vi "Teleop.vi"(10 "Match Info":T1={"Autonomous Elapsed Seconds"=0.72, "TeleOp Elapsed Seconds"=2.218, "Disabled Elapsed Seconds"=2.02, "Visited Autonomous"=TRUE, "Visited TeleOp"=TRUE, "Visited Disabled"=TRUE, "Autonomous Settings"={"Autonomous Style"=enum."Independent", "VI Refnum"=refnum}}, 11 "Call Context":T2=enum."Stop") -> ()   [LabVIEW 2016]
doc: "This VI is called for each TeleOp packet received from the DS where the robot is not disabled. It is often used to read from the joysticks and update I/O or to update setpoints for timed control loops. It should complete and return within 20 milliseconds or it may miss DS packets."
uses:
  <vilib>/Rock Robotics/WPI/DriverStation/WPI_DriverStationDerivedRobotMode.ctl
  <vilib>/Rock Robotics/WPI/DriverStation/WPI_DriverStationMatch Info.ctl
  <vilib>/Rock Robotics/WPI/Utilities/WPI_GetSetVariantRefNum.vi
  Robot Global Data.vi
  <vilib>/Rock Robotics/Network Tables/NT Write Boolean Array.vi
  <vilib>/Rock Robotics/Network Tables/NT Write Numeric Array.vi
  <vilib>/Rock Robotics/Network Tables/NT Read Boolean.vi
  <vilib>/Rock Robotics/Network Tables/NT Read Number.vi
panel:
  in  "Z-axis turn fast":dbl=0.85 format="%#_13g"
  in  "Z-axis turn slow":dbl=0.45 format="%#_13g"
  out "Sample Slider 0":dbl(slide) scale=0.0..5.0
  out "Sample Boolean 1":bool
  out "Sample Boolean 0":bool
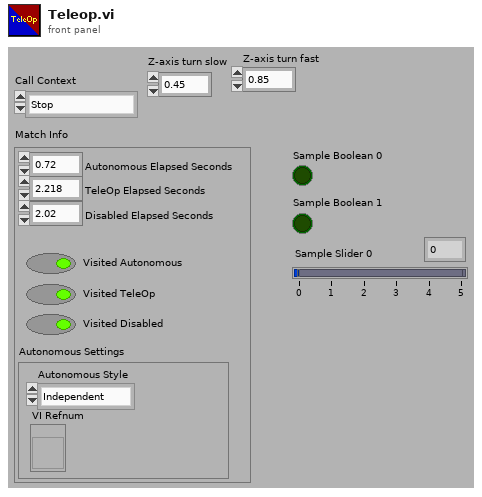
[diagram p1: front panel]
types:
  T1 = typedef "WPI_DriverStationMatch Info.ctl" = cluster{"Autonomous Elapsed Seconds":dbl, "TeleOp Elapsed Seconds":dbl, "Disabled Elapsed Seconds":dbl, "Visited Autonomous":bool, "Visited TeleOp":bool, "Visited Disabled":bool, "Autonomous Settings":cluster{"Autonomous Style":enum16{"Iterative", "Independent"}, "VI Refnum":refnum<vi>}}
  T2 = typedef "WPI_DriverStationDerivedRobotMode.ctl" = enum16{"Init", "Execute", "Stop"}
  T3 = typedef "WPI_JoystickDevRef.ctl" = cluster{"Device":T4}
  T4 = typedef "WPI_JoystickDeviceEnum.ctl" = enum16{"USB 0", "USB 1", "USB 2", "USB 3", "USB 4", "USB 5"}
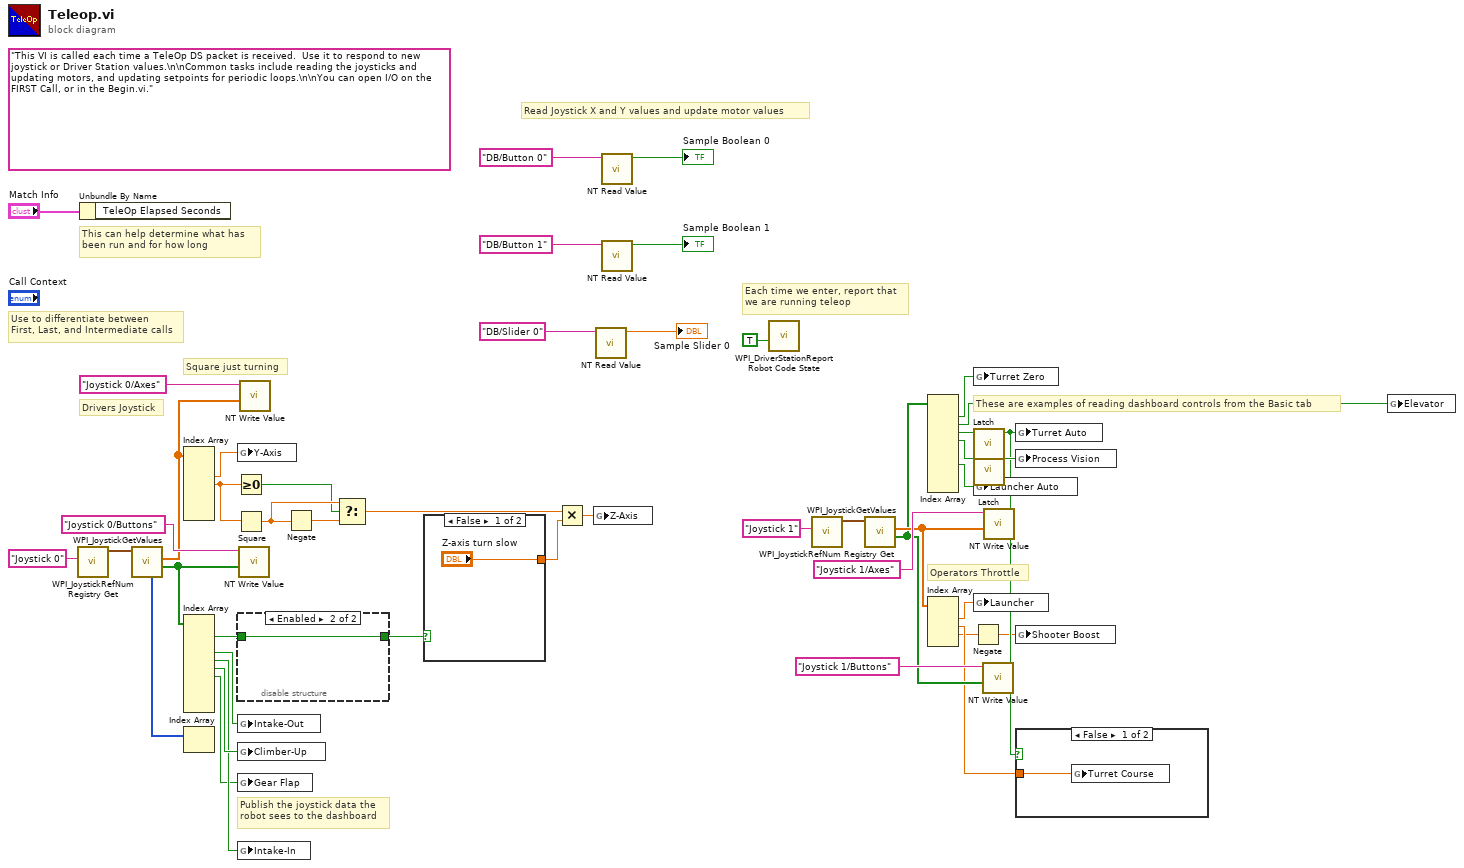
[diagram p0: block diagram]
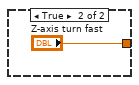
[diagram p2: hidden frame]
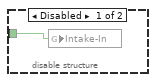
[diagram p3: hidden frame]
diagram:
  (unwired) "This VI is called each time a TeleOp DS packet is received.  Use it to respond to new joystick or Driver Station values.\n\nCommon tasks include reading the joysticks and updating motors, and updating setpoints for periodic loops.\n\nYou can open I/O on the FIRST Call, or in the Begin.vi."
  # "Square just turning"
  # "Drivers Joystick"
  # "Operators Throttle"
  # "These are examples of reading dashboard controls from the Basic tab"
  # "Publish the joystick data the\nrobot sees to the dashboard"
  # "Each time we enter, report that\nwe are running teleop"
  # "Use to differentiate between\nFirst, Last, and Intermediate calls"
  # "This can help determine what has\nbeen run and for how long"
  # "Read Joystick X and Y values and update motor values"
  n1 = call <vilib>:"WPI_JoystickRefNum Registry Get.vi"("refnum name"="Joystick 0") -> ("JoystickDevRef"=w44:T3)  [unwired: 1 in, 9 out]
  n2 = Unbundle By Name("Match Info") -> ()  [unwired: 1 out]
  n3 = call <vilib>:"WPI_JoystickGetValues.vi"("JoystickDevRef"=w44) -> ("Buttons"=w33:bool[], "Axes"=w40:dbl[], "POVs"=w26:i16[])  [unwired: 6 in, 2 out]
  n4 = Index Array(array=w40) -> (element #2=w11:dbl, element #3=w5:dbl)  [unwired: 7 in, 5 out]
  n5 = Index Array(array=w33) -> (element #1=w23:bool, element #3=w1:bool, element #4=w21:bool, element #5=w22:bool, element #6=w20:bool)  [unwired: 10 in, 5 out]
  n6 = Index Array(array=w26) -> ()  [unwired: 1 in, 1 out]
  n7 = Greater Or Equal To 0?(x=w5) -> (x >= 0?=w7:bool)
  n8 = Square(x=w5) -> (x^2=w8:dbl)
  n9 = global write "Robot Global Data.vi" "Y-Axis"(w11) -> ()
  n10 = disable-structure shown="Enabled" {
    disable-tunnel: w23 -> [w47 w48]
    disable-tunnel: [_ w48] -> w3
    frame Disabled {
      n11 = global write "Robot Global Data.vi" "Intake-In"(w47) -> ()
    }
    frame Enabled {
    }
  }
  n12 = global write "Robot Global Data.vi" "Intake-Out"(w1) -> ()
  n13 = global write "Robot Global Data.vi" "Climber-Up"(w22) -> ()
  n14 = global write "Robot Global Data.vi" "Gear Flap"(w20) -> ()
  n15 = global write "Robot Global Data.vi" "Intake-In"(w21) -> ()
  n16 = call-poly <vilib>:"NT Write Value.vi"("Boolean Array"=w33, "Name"="Joystick 0/Buttons") -> ()  [unwired: 9 in, 1 out]
  n17 = call-poly <vilib>:"NT Write Value.vi"("Numeric Array"=w40, "Name"="Joystick 0/Axes") -> ()  [unwired: 9 in, 1 out]
  n18 = Negate(x=w8) -> (-x=w9:dbl)
  n19 = Select(t=w8, s=w7, f=w9) -> (s? t:f=w6:dbl)
  n20 = case shown="False" w3 {
    tunnel: ["Z-axis turn slow" "Z-axis turn fast"] -> w10
    frame False {
    }
    frame True {
    }
  }
  n21 = Multiply(x=w6, y=w10) -> (x*y=w4:dbl)
  n22 = global write "Robot Global Data.vi" "Z-Axis"(w4) -> ()
  n23 = call-poly <vilib>:"NT Read Value.vi"("Name"="DB/Slider 0" ("refnum name")) -> ("Numeric"=→"Sample Slider 0":dbl)  [unwired: 9 in, 1 out]
  n24 = call-poly <vilib>:"NT Read Value.vi"("Name"="DB/Button 0" ("refnum name")) -> ("Boolean"=→"Sample Boolean 0":bool)  [unwired: 9 in, 1 out]
  n25 = call-poly <vilib>:"NT Read Value.vi"("Name"="DB/Button 1" ("refnum name")) -> ("Boolean"=→"Sample Boolean 1":bool)  [unwired: 9 in, 1 out]
  n26 = call <vilib>:"WPI_DriverStationReport Robot Code State.vi"("TeleOp"=TRUE ("Autonomous")) -> ()  [unwired: 10 in, 1 out]
  n27 = call <vilib>:"WPI_JoystickRefNum Registry Get.vi"("refnum name"="Joystick 1") -> ("JoystickDevRef"=w31:T3)  [unwired: 1 in, 9 out]
  n28 = call <vilib>:"WPI_JoystickGetValues.vi"("JoystickDevRef"=w31) -> ("Buttons"=w27:bool[], "Axes"=w28:dbl[])  [unwired: 6 in, 3 out]
  n29 = Index Array(array=w27) -> (element #1=w24:bool, element #2=w2:bool, element #3=w19:bool, element #4=w18:bool, element #7=w12:bool)  [unwired: 10 in, 5 out]
  n30 = Index Array(array=w28) -> (element #1=w15:dbl, element #2=w25:dbl, element #3=w14:dbl)  [unwired: 4 in, 1 out]
  n31 = Negate(x=w14) -> (-x=w13:dbl)
  n32 = global write "Robot Global Data.vi" "Turret Zero"(w24) -> ()
  n33 = call "Latch.vi"("In"=w19) -> ("Out"=w16:bool)  [unwired: 9 in, 1 out]
  n34 = call "Latch.vi"("In"=w18) -> ("Out"=w17:bool)  [unwired: 9 in, 1 out]
  n35 = global write "Robot Global Data.vi" "Launcher Auto"(w12) -> ()
  n36 = global write "Robot Global Data.vi" "Launcher"(w15) -> ()
  n37 = call-poly <vilib>:"NT Write Value.vi"("Boolean Array"=w27, "Name"="Joystick 1/Buttons") -> ()  [unwired: 9 in, 1 out]
  n38 = call-poly <vilib>:"NT Write Value.vi"("Numeric Array"=w28, "Name"="Joystick 1/Axes") -> ()  [unwired: 9 in, 1 out]
  n39 = global write "Robot Global Data.vi" "Turret Auto"(w16) -> ()
  n40 = global write "Robot Global Data.vi" "Process Vision"(w17) -> ()
  n41 = global write "Robot Global Data.vi" "Shooter Boost"(w13) -> ()
  n42 = case shown="False" w16 {
    tunnel: w25 -> [w51 _]
    frame False {
      n43 = global write "Robot Global Data.vi" "Turret Course"(w51) -> ()
    }
    frame True {
    }
  }
  n44 = global write "Robot Global Data.vi" "Elevator"(w2) -> ()
